vi "ExecutePlay.vi"(0 "object in":refnum<class "Play_v2.lvclass">, 2 "Robots in":refnum<class "Robot.lvclass">[](array[class]), 3 "GameRef":refnum<data-value>, 5 "error in (no error)":errorcluster) -> (14 "object out":refnum<class "Play_v2.lvclass">, 16 "Robots out":refnum<class "Robot.lvclass">[](array[class]), 19 "error out":errorcluster)   [LabVIEW 2023, in "Play_v2.lvclass"]
uses:
  Play_v2.lvclass
  Robot_class/Robot.lvclass
  Game_class/Game.lvclass
  NewRoles/Role_v2_class/Role_v2.lvclass
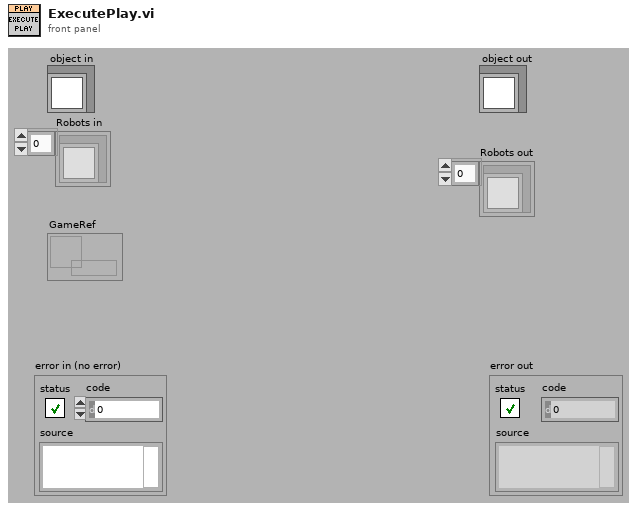
[diagram p1: front panel]
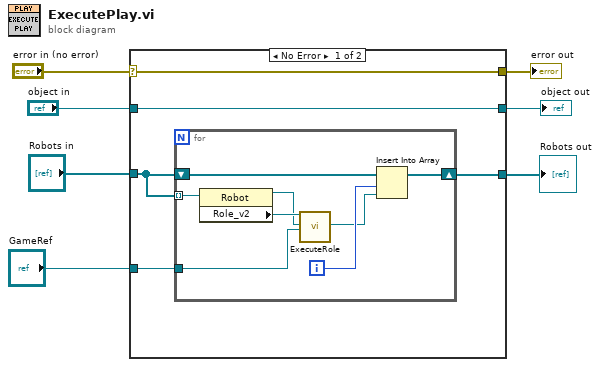
[diagram p0: block diagram]
diagram:
  n1 = case shown="No Error" "error in (no error)" {
    selector: "error in (no error)" -> [w12 w23]
    tunnel: [w12 w23] -> w6
    tunnel: [w11 w22] -> w4
    tunnel: "object in" -> [w11 w22]
    tunnel: "Robots in" -> [w10 w21]
    tunnel: [w9 w21] -> w2
    tunnel: "GameRef" -> [w8 _]
    frame No Error {
      n2 = for {
        tunnel: w10 -> [w20] mode=indexing
        shift-right: [w14] -> w9
        shift-left: w10 -> [w15]
        tunnel: w8 -> [w13]
        i -> [w17]
        n3 = property class="Robot"(reference=w20) -> (reference out=w18:refnum<class "Robot.lvclass">, "Role_v2"=w19:refnum<class "Role_v2.lvclass">)  [unwired: 1 in, 1 out]
        n4 = call-dynamic "ExecuteRole.vi"("object in"=w19, "Robot in"=w18, "GameRef"=w13) -> ("Robot out"=w16:refnum<class "Robot.lvclass">)  [unwired: 14 in, 2 out]
        n5 = Insert Into Array(array=w15, index=w17, new element=w16) -> (w14:refnum<class "Robot.lvclass">[])
      }
    }
    frame Error {
    }
  }
  "error out" <- w6
  "object out" <- w4
  "Robots out" <- w2
